vi "Builder.Set Interface.vi"(10 "Builder Interface":refnum<class "DSF.Engine.Interface.Builder.lvclass">, 11 "Builder in":refnum<class "Builder.lvclass">) -> (3 "Builder out":refnum<class "Builder.lvclass">)   [LabVIEW 2016, in "DSF.Engine.lvlib" / "Builder.lvclass"]
uses:
  Builder.lvclass
  Interface/DSF.Engine.Interface.Builder.lvclass
  Builder.lvclass/Builder.ctl
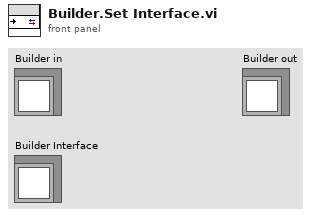
[diagram p1: front panel]
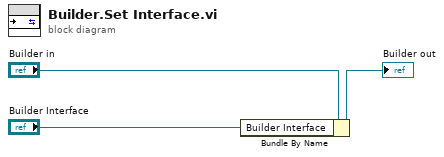
[diagram p0: block diagram]
diagram:
  n1 = Bundle By Name(cluster="Builder in", "Builder Interface"="Builder Interface") -> (→"Builder out":refnum<class "Builder.lvclass">)
